vi "Throttle.vi"() -> ()   [LabVIEW 2018]
panel:
  in  "File Tag":string
  out "Data Log":bool
  out "Auto Started":bool
  in  "Alarm Action":string
  out "dATA_BOOL":bool[](array[boolean])
  in  "rpm torque":dbl[](array[numeric])
  in  "DAT DOUBLE":dbl[](array[numeric])
  out "Throttle %":fxp<+/-,34,12>
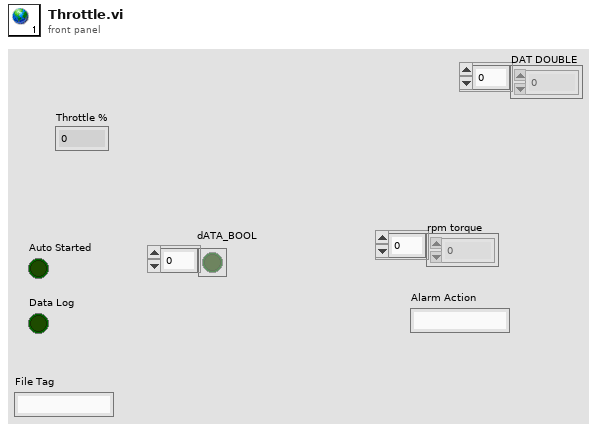
[diagram p1: front panel]
diagram:
